vi "CheckInterlocks.vi"(0 "Interlock Array":T1) -> (1 "Failed Interlock List":string[](array[string]), 2 "All Ready?":bool=TRUE, 3 "Numer Of Failures":i32)   [LabVIEW 2016]
uses:
  InterlockArray.ctl
  InterlockElement.ctl
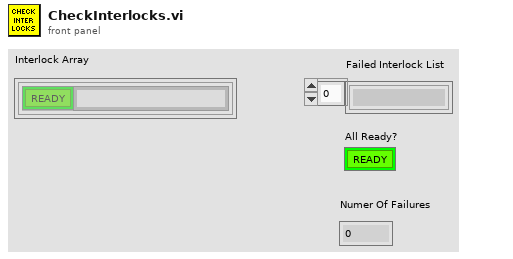
[diagram p1: front panel]
types:
  T1 = typedef "InterlockArray.ctl" = T2[]
  T2 = typedef "InterlockElement.ctl" = cluster{"Interlock State":bool, "Interlock Name":string}
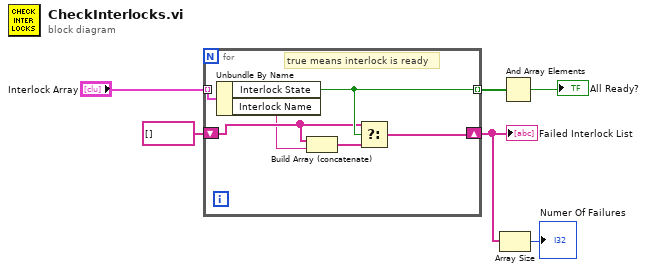
[diagram p0: block diagram]
diagram:
  n1 = for {
    tunnel: "Interlock Array" -> [w12] mode=indexing
    tunnel: [w11] -> w4 mode=indexing
    shift-right: [w10] -> w2
    shift-left: string[] [] -> [w9]
    # "true means interlock is ready"
    n2 = Unbundle By Name(w12) -> ("Interlock State"=w11:bool, "Interlock Name"=w8:string)
    n3 = Build Array (concatenate)(w9, w8) -> (w7:string[])
    n4 = Select(t=w9, s=w11, f=w7) -> (s? t:f=w10:string[])
  }
  "Failed Interlock List" <- w2
  n5 = Array Size(array=w2) -> (size(s)=→"Numer Of Failures":i32)
  n6 = And Array Elements(Boolean array=w4) -> (logical AND=→"All Ready?":bool)
